vi "Ask User For Import CSV File Location.vi"(8 "error in (no error)":errorcluster) -> (0 "error out":errorcluster, 2 "cancelled":bool, 3 "selected path":path)   [LabVIEW 2019, in "Diagnostics Addon System Explorer.lvlib"]
uses:
  Diagnostics Addon System Explorer.lvlib
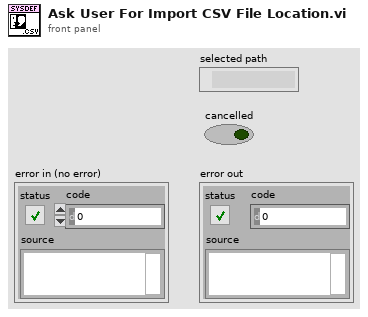
[diagram p1: front panel]
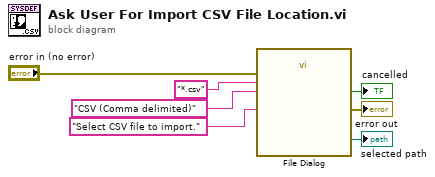
[diagram p0: block diagram]
diagram:
  n1 = call "File Dialog"("prompt"="Select CSV file to import.", "error in"="error in (no error)", "pattern (all files)"="*.csv" ("pattern label"), "pattern label"="CSV (Comma delimited)") -> ("selected path"=→"selected path":path, "cancelled"=→"cancelled":bool, "error out"=→"error out":errorcluster)  [unwired: 8 in, 1 out]
